vi "Set Server Stop UE.vi"(10 "Server Stop UE":refnum<user-event>, 11 "OOP Server in":refnum<class "helloWServer.lvclass">) -> (3 "OOP Server out":refnum<class "helloWServer.lvclass">)   [LabVIEW 2020, in "helloWServer.lvlib" / "helloWServer.lvclass"]
uses:
  helloWServer.lvclass
  helloWServer.lvclass/helloWServer.ctl
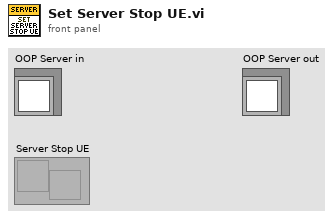
[diagram p1: front panel]
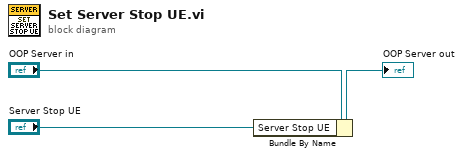
[diagram p0: block diagram]
diagram:
  n1 = Bundle By Name(cluster="OOP Server in", "Server Stop UE"="Server Stop UE") -> (→"OOP Server out":refnum<class "helloWServer.lvclass">)
